vi "Repartidor_colores.vi"() -> ()   [LabVIEW 2017]
uses:
  <extravilib>/ChannelInstances/Stream-bool/Read With Abort.vi
  <extravilib>/ChannelInstances/Stream-bool/Write With Abort.vi
  <extravilib>/ChannelInstances/Stream-bool/EndpointRead.vi
  <extravilib>/ChannelInstances/Stream-bool/Endpoint.vi
  <extravilib>/ChannelInstances/Stream-bool/Instantiate.vi
  <extravilib>/ChannelInstances/Stream-bool/)Channel.vi
  <resource>/ChannelSupport/_ChannelSupport/WaitIfNeeded.vi
  <extravilib>/ChannelInstances/Stream-bool.lvlib
panel:
  out "A 10":u32[][](array[colorbox])
  out "A 9":u32[][](array[colorbox])
  out "A 8":u32[][](array[colorbox])
  out "A 7":u32[][](array[colorbox])
  out "A 6":u32[][](array[colorbox])
  out "A 5":u32[][](array[colorbox])
  out "A 4":u32[][](array[colorbox])
  out "A 3":u32[][](array[colorbox])
  out "A 2":u32[][](array[colorbox])
  out "A":u32[][](array[colorbox])
  out "Array 4":u32[](array[numeric])
  out "element 2":u32
  in  "stop":bool
  out "element":u32
  out "Color Box":u32(colorbox)
  out "Array 2":u32[](array[colorbox])
  out "Array":u32[][](array[colorbox])
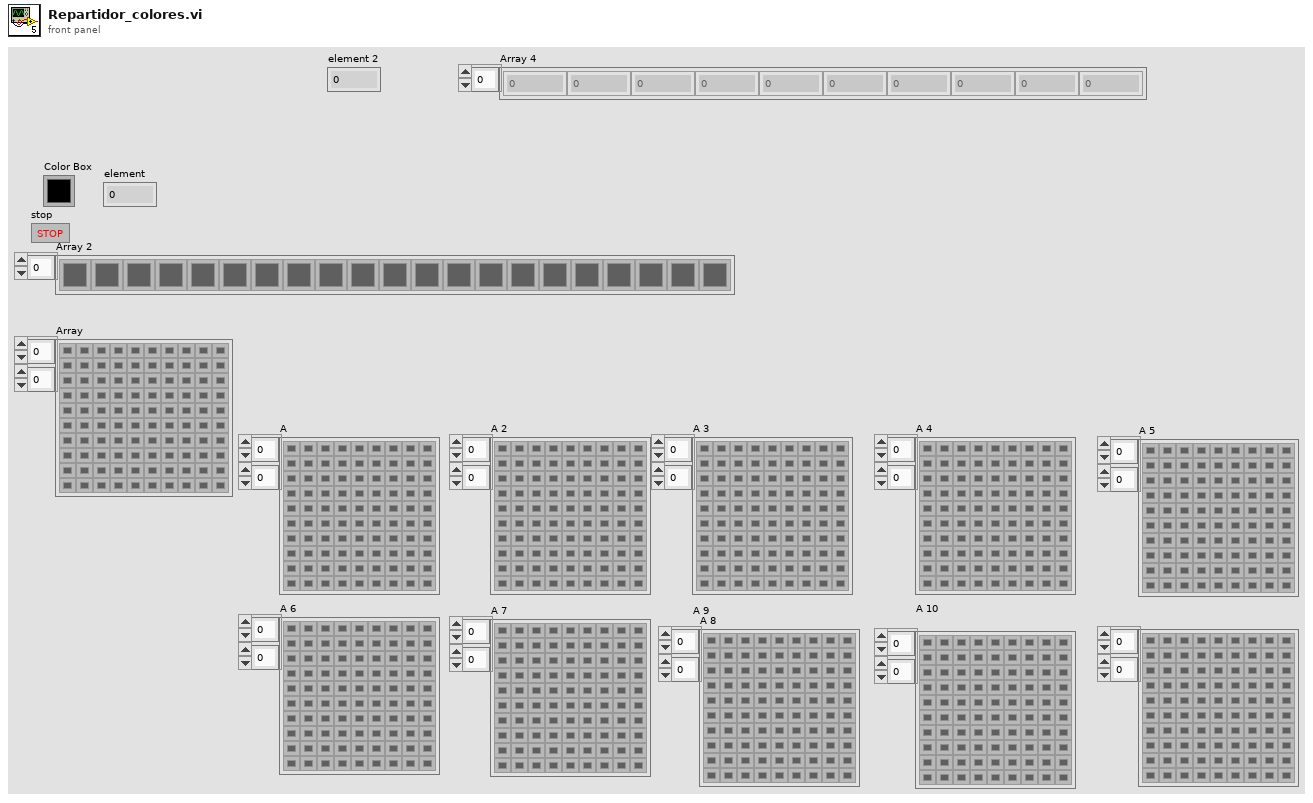
[diagram p1: front panel]
types:
  T1 = cluster{"Numeros":u32[], "A1":u32[], "B1":u32[], "C1":u32[], "D1":u32[], "E1":u32[], "F1":u32[], "G1":u32[], "H1":u32[], "I1":u32[], "J1":u32[]}
  T2 = typedef "Stream-bool.lvlib/)Channel.ctl" = refnum<queue>
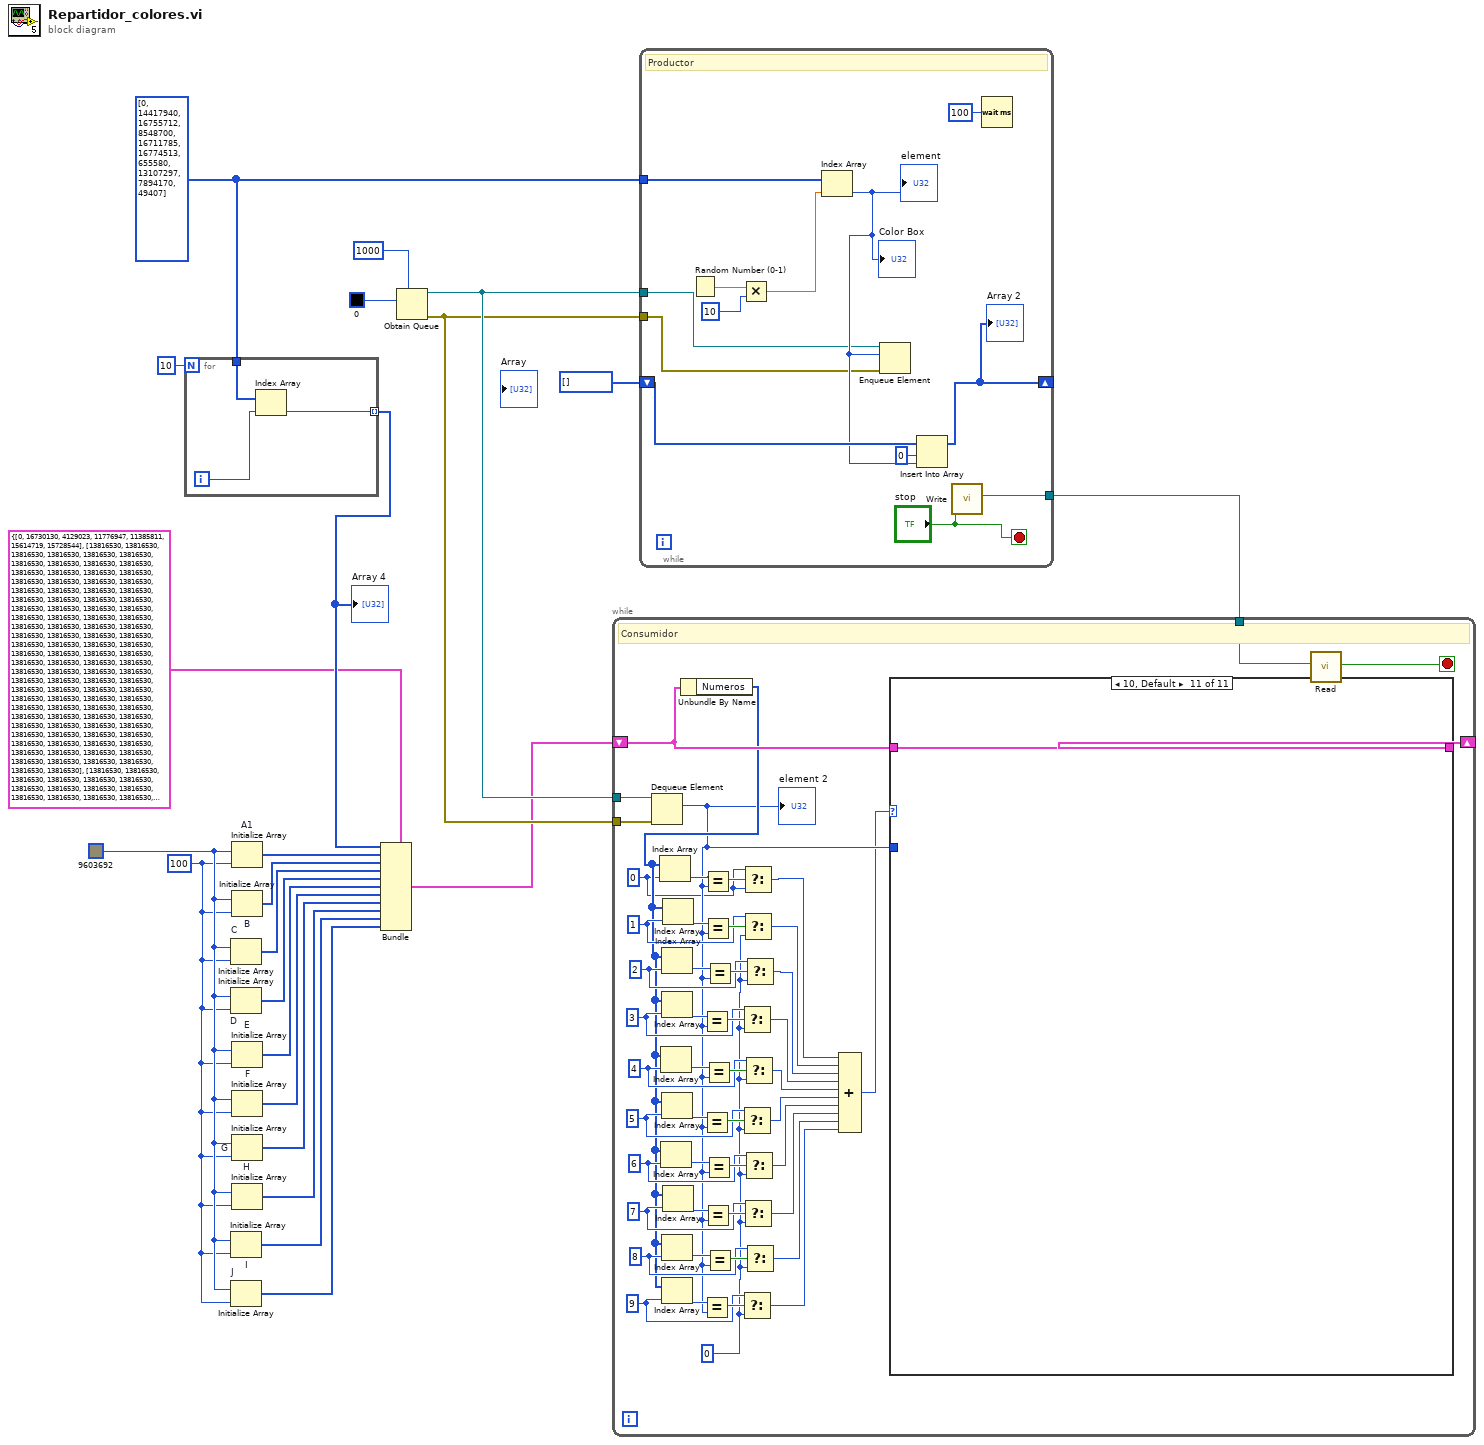
[diagram p0: block diagram]
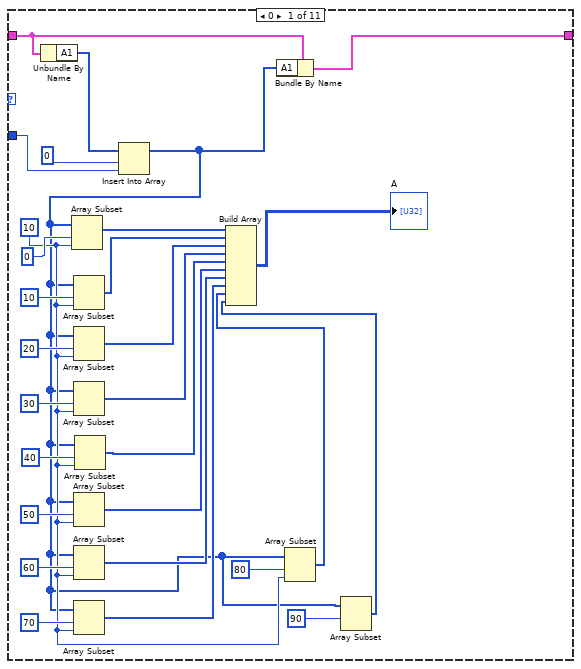
[diagram p2: hidden frame]
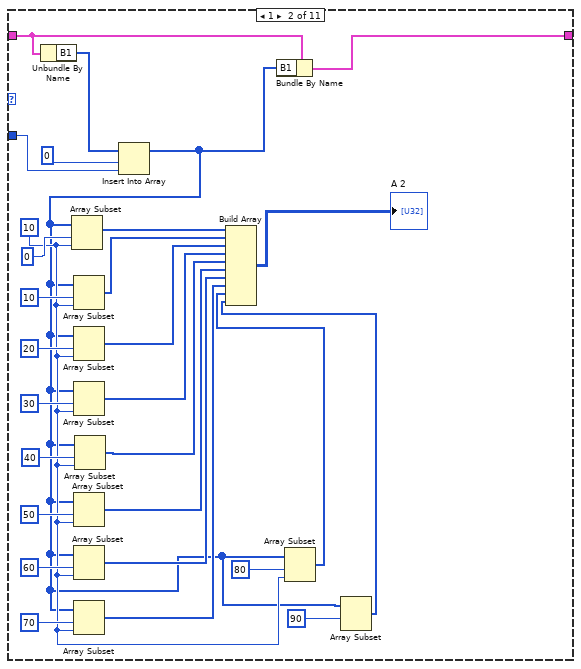
[diagram p3: hidden frame]
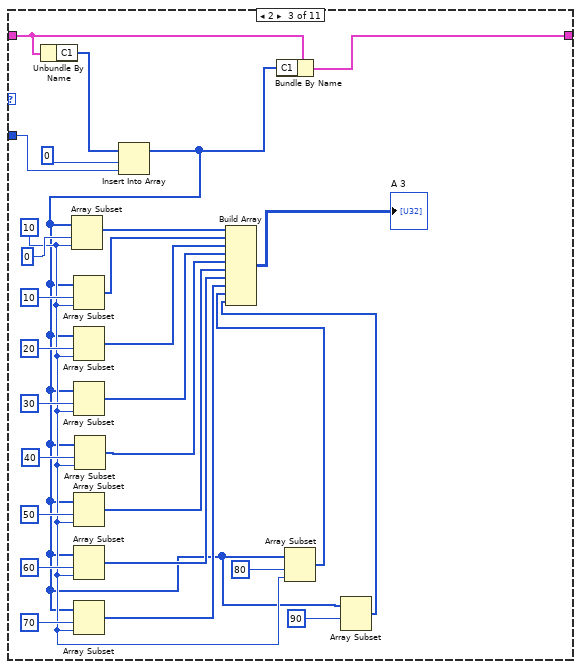
[diagram p4: hidden frame]
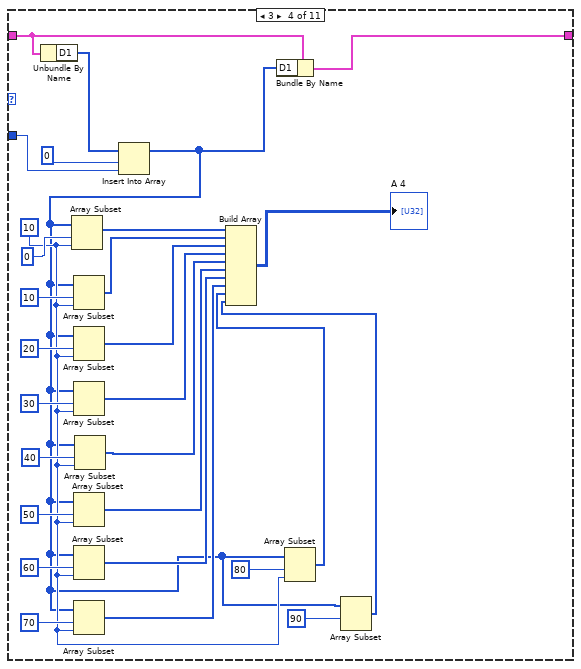
[diagram p5: hidden frame]
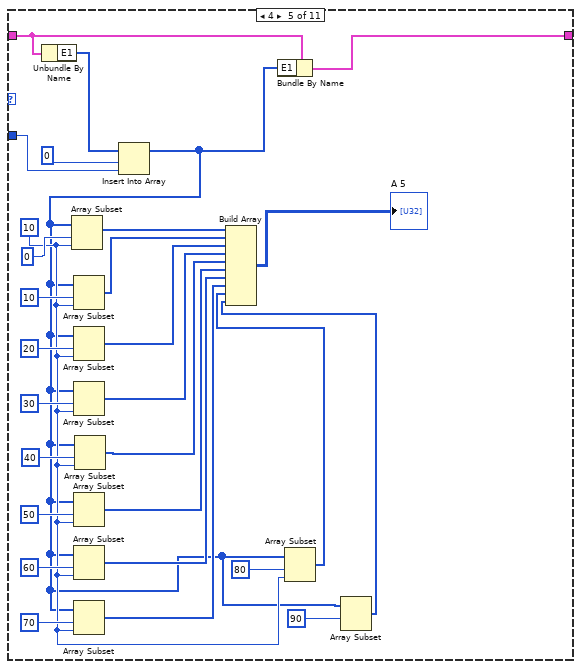
[diagram p6: hidden frame]
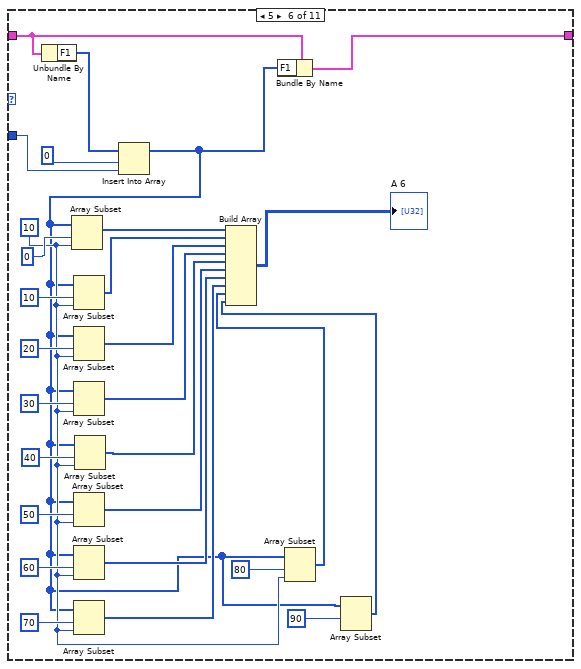
[diagram p7: hidden frame]
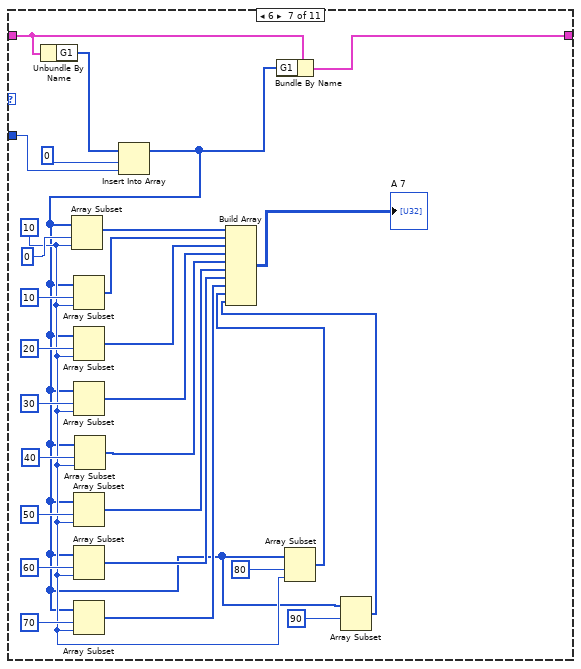
[diagram p8: hidden frame]
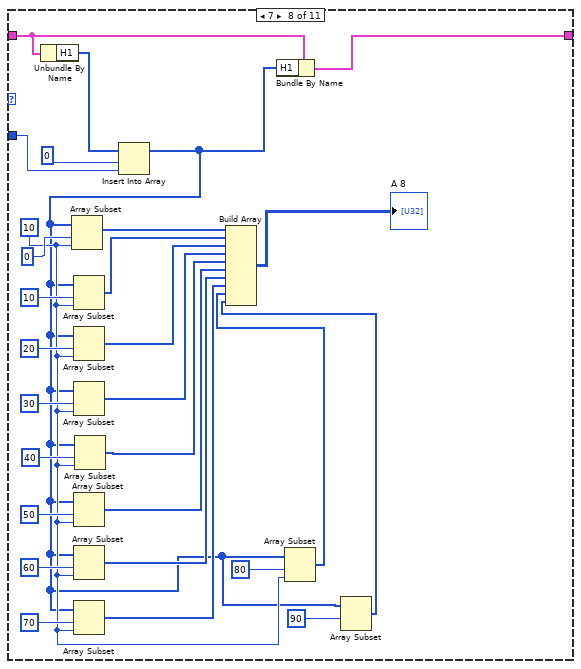
[diagram p9: hidden frame]
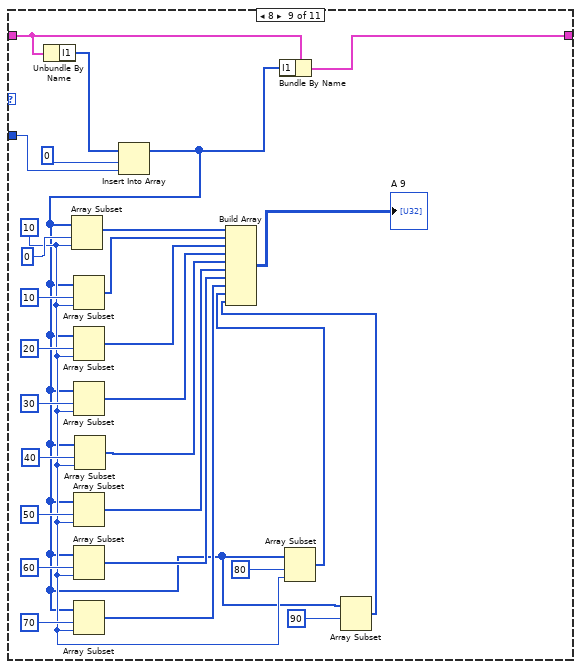
[diagram p10: hidden frame]
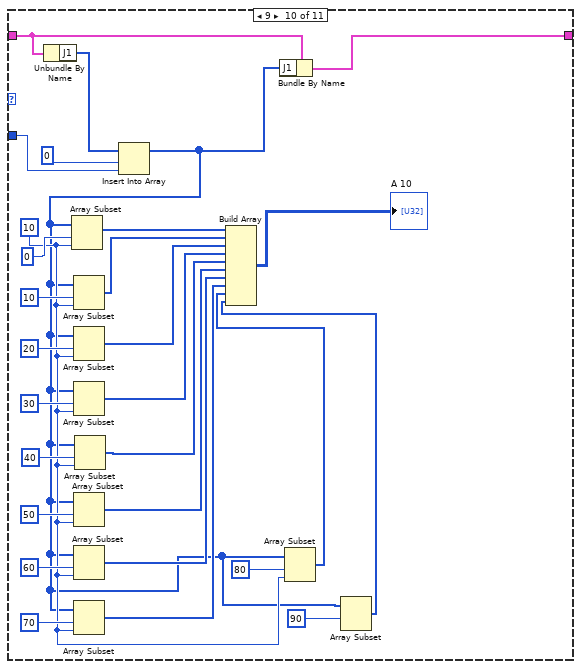
[diagram p11: hidden frame]
diagram:
  w2 = u32[] [0, 14417940, 16755712, 8548700, 16711785, 16774513, 655580, 13107297, 7894170, 49407]
  w18 = u32 9603692
  w17 = 100 ("dimension size")
  n1 = for {
    N: 10 -> [_]
    tunnel: w2 -> [w26]
    tunnel: [w24] -> w7 mode=indexing
    i -> [w25]
    n2 = Index Array "Index Array"(array=w26, index=w25) -> (element=w24:u32)
  }
  "Array 4" <- w7
  n3 = Initialize Array "C"(w18, w17) -> (w16:u32[])
  n4 = Initialize Array "D"(w18, w17) -> (w15:u32[])
  n5 = Initialize Array "I"(w18, w17) -> (w10:u32[])
  n6 = Initialize Array "J"(w18, w17) -> (w9:u32[])
  n7 = Initialize Array "A1"(w18, w17) -> (w5:u32[])
  n8 = Initialize Array "B"(w18, w17) -> (w6:u32[])
  n9 = Initialize Array "E"(w18, w17) -> (w14:u32[])
  n10 = Initialize Array "F"(w18, w17) -> (w13:u32[])
  n11 = Initialize Array "G"(w18, w17) -> (w12:u32[])
  n12 = Initialize Array "H"(w18, w17) -> (w11:u32[])
  n13 = Bundle "Bundle"(cluster=T1 {"Numeros"=[0, 16730130, 4129023, 11776947, 11385811, 15614719, 15728544], "A1"=[13816530, 13816530, 13816530, 13816530, 13816530, 13816530, 13816530, 13816530, 13816530, 13816530, 13816530, 13816530, 13816530, 13816530, 13816530, 13816530, 13816530, 13816530, 13816530, 13816530, 13816530, 13816530, 13816530, 13816530, 13816530, 13816530, 13816530, 13816530, 13816530, 13816530, 13816530, 13816530, 13816530, 13816530, 13816530, 13816530, 13816530, 13816530, 13816530, 13816530, 13816530, 13816530, 13816530, 13816530, 13816530, 13816530, 13816530, 13816530, 13816530, 13816530, 13816530, 13816530, 13816530, 13816530, 13816530, 13816530, 13816530, 13816530, 13816530, 13816530, 13816530, 13816530, 13816530, 13816530, 13816530, 13816530, 13816530, 13816530, 13816530, 13816530, 13816530, 13816530, 13816530, 13816530, 13816530, 13816530, 13816530, 13816530, 13816530, 13816530, 13816530, 13816530, 13816530, 13816530, 13816530, 13816530, 13816530, 13816530, 13816530, 13816530, 13816530, 13816530, 13816530, 13816530, 13816530, 13816530, 13816530, 13816530, 13816530, 13816530], "B1"=[13816530, 13816530, 13816530, 13816530, 13816530, 13816530, 13816530, 13816530, 13816530, 13816530, 13816530, 13816530, 13816530, 13816530, 13816530, 13816530, 13816530, 13816530, 13816530, 13816530, 13816530, 13816530, 13816530, 13816530, 13816530, 13816530, 13816530, 13816530, 13816530, 13816530, 13816530, 13816530, 13816530, 13816530, 13816530, 13816530, 13816530, 13816530, 13816530, 13816530, 13816530, 13816530, 13816530, 13816530, 13816530, 13816530, 13816530, 13816530, 13816530, 13816530, 13816530, 13816530, 13816530, 13816530, 13816530, 13816530, 13816530, 13816530, 13816530, 13816530, 13816530, 13816530, 13816530, 13816530, 13816530, 13816530, 13816530, 13816530, 13816530, 13816530, 13816530, 13816530, 13816530, 13816530, 13816530, 13816530, 13816530, 13816530, 13816530, 13816530, 13816530, 13816530, 13816530, 13816530, 13816530, 13816530, 13816530, 13816530, 13816530, 13816530, 13816530, 13816530, 13816530, 13816530, 13816530, 13816530, 13816530, 13816530, 13816530, 13816530], "C1"=[13816530, 13816530, 13816530, 13816530, 13816530, 13816530, 13816530, 13816530, 13816530, 13816530, 13816530, 13816530, 13816530, 13816530, 13816530, 13816530, 13816530, 13816530, 13816530, 13816530, 13816530, 13816530, 13816530, 13816530, 13816530, 13816530, 13816530, 13816530, 13816530, 13816530, 13816530, 13816530, 13816530, 13816530, 13816530, 13816530, 13816530, 13816530, 13816530, 13816530, 13816530, 13816530, 13816530, 13816530, 13816530, 13816530, 13816530, 13816530, 13816530, 13816530, 13816530, 13816530, 13816530, 13816530, 13816530, 13816530, 13816530, 13816530, 13816530, 13816530, 13816530, 13816530, 13816530, 13816530, 13816530, 13816530, 13816530, 13816530, 13816530, 13816530, 13816530, 13816530, 13816530, 13816530, 13816530, 13816530, 13816530, 13816530, 13816530, 13816530, 13816530, 13816530, 13816530, 13816530, 13816530, 13816530, 13816530, 13816530, 13816530, 13816530, 13816530, 13816530, 13816530, 13816530, 13816530, 13816530, 13816530, 13816530, 13816530, 13816530], "D1"=[13816530, 13816530, 13816530, 13816530, 13816530, 13816530, 13816530, 13816530, 13816530, 13816530, 13816530, 13816530, 13816530, 13816530, 13816530, 13816530, 13816530, 13816530, 13816530, 13816530, 13816530, 13816530, 13816530, 13816530, 13816530, 13816530, 13816530, 13816530, 13816530, 13816530, 13816530, 13816530, 13816530, 13816530, 13816530, 13816530, 13816530, 13816530, 13816530, 13816530, 13816530, 13816530, 13816530, 13816530, 13816530, 13816530, 13816530, 13816530, 13816530, 13816530, 13816530, 13816530, 13816530, 13816530, 13816530, 13816530, 13816530, 13816530, 13816530, 13816530, 13816530, 13816530, 13816530, 13816530, 13816530, 13816530, 13816530, 13816530, 13816530, 13816530, 13816530, 13816530, 13816530, 13816530, 13816530, 13816530, 13816530, 13816530, 13816530, 13816530, 13816530, 13816530, 13816530, 13816530, 13816530, 13816530, 13816530, 13816530, 13816530, 13816530, 13816530, 13816530, 13816530, 13816530, 13816530, 13816530, 13816530, 13816530, 13816530, 13816530], "E1"=[13816530, 13816530, 13816530, 13816530, 13816530, 13816530, 13816530, 13816530, 13816530, 13816530, 13816530, 13816530, 13816530, 13816530, 13816530, 13816530, 13816530, 13816530, 13816530, 13816530, 13816530, 13816530, 13816530, 13816530, 13816530, 13816530, 13816530, 13816530, 13816530, 13816530, 13816530, 13816530, 13816530, 13816530, 13816530, 13816530, 13816530, 13816530, 13816530, 13816530, 13816530, 13816530, 13816530, 13816530, 13816530, 13816530, 13816530, 13816530, 13816530, 13816530, 13816530, 13816530, 13816530, 13816530, 13816530, 13816530, 13816530, 13816530, 13816530, 13816530, 13816530, 13816530, 13816530, 13816530, 13816530, 13816530, 13816530, 13816530, 13816530, 13816530, 13816530, 13816530, 13816530, 13816530, 13816530, 13816530, 13816530, 13816530, 13816530, 13816530, 13816530, 13816530, 13816530, 13816530, 13816530, 13816530, 13816530, 13816530, 13816530, 13816530, 13816530, 13816530, 13816530, 13816530, 13816530, 13816530, 13816530, 13816530, 13816530, 13816530], "F1"=[13816530, 13816530, 13816530, 13816530, 13816530, 13816530, 13816530, 13816530, 13816530, 13816530, 13816530, 13816530, 13816530, 13816530, 13816530, 13816530, 13816530, 13816530, 13816530, 13816530, 13816530, 13816530, 13816530, 13816530, 13816530, 13816530, 13816530, 13816530, 13816530, 13816530, 13816530, 13816530, 13816530, 13816530, 13816530, 13816530, 13816530, 13816530, 13816530, 13816530, 13816530, 13816530, 13816530, 13816530, 13816530, 13816530, 13816530, 13816530, 13816530, 13816530, 13816530, 13816530, 13816530, 13816530, 13816530, 13816530, 13816530, 13816530, 13816530, 13816530, 13816530, 13816530, 13816530, 13816530, 13816530, 13816530, 13816530, 13816530, 13816530, 13816530, 13816530, 13816530, 13816530, 13816530, 13816530, 13816530, 13816530, 13816530, 13816530, 13816530, 13816530, 13816530, 13816530, 13816530, 13816530, 13816530, 13816530, 13816530, 13816530, 13816530, 13816530, 13816530, 13816530, 13816530, 13816530, 13816530, 13816530, 13816530, 13816530, 13816530], "G1"=[13816530, 13816530, 13816530, 13816530, 13816530, 13816530, 13816530, 13816530, 13816530, 13816530, 13816530, 13816530, 13816530, 13816530, 13816530, 13816530, 13816530, 13816530, 13816530, 13816530, 13816530, 13816530, 13816530, 13816530, 13816530, 13816530, 13816530, 13816530, 13816530, 13816530, 13816530, 13816530, 13816530, 13816530, 13816530, 13816530, 13816530, 13816530, 13816530, 13816530, 13816530, 13816530, 13816530, 13816530, 13816530, 13816530, 13816530, 13816530, 13816530, 13816530, 13816530, 13816530, 13816530, 13816530, 13816530, 13816530, 13816530, 13816530, 13816530, 13816530, 13816530, 13816530, 13816530, 13816530, 13816530, 13816530, 13816530, 13816530, 13816530, 13816530, 13816530, 13816530, 13816530, 13816530, 13816530, 13816530, 13816530, 13816530, 13816530, 13816530, 13816530, 13816530, 13816530, 13816530, 13816530, 13816530, 13816530, 13816530, 13816530, 13816530, 13816530, 13816530, 13816530, 13816530, 13816530, 13816530, 13816530, 13816530, 13816530, 13816530], "H1"=[13816530, 13816530, 13816530, 13816530, 13816530, 13816530, 13816530, 13816530, 13816530, 13816530, 13816530, 13816530, 13816530, 13816530, 13816530, 13816530, 13816530, 13816530, 13816530, 13816530, 13816530, 13816530, 13816530, 13816530, 13816530, 13816530, 13816530, 13816530, 13816530, 13816530, 13816530, 13816530, 13816530, 13816530, 13816530, 13816530, 13816530, 13816530, 13816530, 13816530, 13816530, 13816530, 13816530, 13816530, 13816530, 13816530, 13816530, 13816530, 13816530, 13816530, 13816530, 13816530, 13816530, 13816530, 13816530, 13816530, 13816530, 13816530, 13816530, 13816530, 13816530, 13816530, 13816530, 13816530, 13816530, 13816530, 13816530, 13816530, 13816530, 13816530, 13816530, 13816530, 13816530, 13816530, 13816530, 13816530, 13816530, 13816530, 13816530, 13816530, 13816530, 13816530, 13816530, 13816530, 13816530, 13816530, 13816530, 13816530, 13816530, 13816530, 13816530, 13816530, 13816530, 13816530, 13816530, 13816530, 13816530, 13816530, 13816530, 13816530], "I1"=[13816530, 13816530, 13816530, 13816530, 13816530, 13816530, 13816530, 13816530, 13816530, 13816530, 13816530, 13816530, 13816530, 13816530, 13816530, 13816530, 13816530, 13816530, 13816530, 13816530, 13816530, 13816530, 13816530, 13816530, 13816530, 13816530, 13816530, 13816530, 13816530, 13816530, 13816530, 13816530, 13816530, 13816530, 13816530, 13816530, 13816530, 13816530, 13816530, 13816530, 13816530, 13816530, 13816530, 13816530, 13816530, 13816530, 13816530, 13816530, 13816530, 13816530, 13816530, 13816530, 13816530, 13816530, 13816530, 13816530, 13816530, 13816530, 13816530, 13816530, 13816530, 13816530, 13816530, 13816530, 13816530, 13816530, 13816530, 13816530, 13816530, 13816530, 13816530, 13816530, 13816530, 13816530, 13816530, 13816530, 13816530, 13816530, 13816530, 13816530, 13816530, 13816530, 13816530, 13816530, 13816530, 13816530, 13816530, 13816530, 13816530, 13816530, 13816530, 13816530, 13816530, 13816530, 13816530, 13816530, 13816530, 13816530, 13816530, 13816530], "J1"=[13816530, 13816530, 13816530, 13816530, 13816530, 13816530, 13816530, 13816530, 13816530, 13816530, 13816530, 13816530, 13816530, 13816530, 13816530, 13816530, 13816530, 13816530, 13816530, 13816530, 13816530, 13816530, 13816530, 13816530, 13816530, 13816530, 13816530, 13816530, 13816530, 13816530, 13816530, 13816530, 13816530, 13816530, 13816530, 13816530, 13816530, 13816530, 13816530, 13816530, 13816530, 13816530, 13816530, 13816530, 13816530, 13816530, 13816530, 13816530, 13816530, 13816530, 13816530, 13816530, 13816530, 13816530, 13816530, 13816530, 13816530, 13816530, 13816530, 13816530, 13816530, 13816530, 13816530, 13816530, 13816530, 13816530, 13816530, 13816530, 13816530, 13816530, 13816530, 13816530, 13816530, 13816530, 13816530, 13816530, 13816530, 13816530, 13816530, 13816530, 13816530, 13816530, 13816530, 13816530, 13816530, 13816530, 13816530, 13816530, 13816530, 13816530, 13816530, 13816530, 13816530, 13816530, 13816530, 13816530, 13816530, 13816530, 13816530, 13816530]}, "Numeros"=w7, "A1"=w5, "B1"=w6, "C1"=w16, "D1"=w15, "E1"=w14, "F1"=w13, "G1"=w12, "H1"=w11, "I1"=w10, "J1"=w9) -> (w4:T1)
  n14 = Obtain Queue(max queue size (-1, unlimited)=1000, element data type=u32 0) -> (queue out=w20:refnum<queue>, error out=w19:errorcluster)  [unwired: 3 in, 1 out]
  n15 = while {
    shift-right: [w32] -> _
    shift-left: u32[] [] -> [w34]
    tunnel: w19 -> [w30]
    tunnel: w20 -> [w29]
    tunnel: w2 -> [w28]
    tunnel: [w27] -> w1
    stop <- "stop" stop-if-true
    # "Productor"
    n16 = Random Number (0-1)() -> (number: 0 to 1=w39:dbl)
    n17 = Multiply(x=w39, y=10) -> (x*y=w37:dbl)
    n18 = Index Array "Index Array"(array=w28, index=w37) -> (element=w31:u32)
    "element" <- w31
    "Color Box" <- w31
    n19 = Enqueue Element(queue=w29, element=w31, error in (no error)=w30) -> ()  [unwired: 1 in, 3 out]
    n20 = Insert Into Array "Insert Into Array"(array=w34, index=0, new element=w31) -> (w32:u32[])
    "Array 2" <- w32
    n21 = call <extravilib>:"Write.vi"("element"="stop") -> ("channel"=w27:T2)  [unwired: 8 in, 2 out]
    n22 = Wait (ms)(milliseconds to wait=u32 100) -> ()  [unwired: 1 out]
  }
  n23 = while {
    tunnel: w20 -> [w89]
    tunnel: w19 -> [w88]
    shift-right: [w87] -> _
    shift-left: w4 -> [w86]
    tunnel: w1 -> [w41]
    stop <- w40 stop-if-true
    w43 = 0 ("f")
    w66 = 9 ("index")
    w68 = 8 ("index")
    w70 = 7 ("index")
    w72 = 6 ("index")
    w74 = 5 ("index")
    w76 = 4 ("index")
    w78 = 3 ("index")
    w80 = 2 ("index")
    w82 = 1 ("index")
    w54 = 0 ("index")
    # "Consumidor"
    n24 = Dequeue Element(queue=w89, error in (no error)=w88) -> (element=w55:u32)  [unwired: 1 in, 3 out]
    "element 2" <- w55
    n25 = Unbundle By Name(w86) -> ("Numeros"=w65:u32[])
    n26 = Index Array(array=w65, index=w54) -> (element=w85:u32)
    n27 = Index Array(array=w65, index=w76) -> (element=w59:u32)
    n28 = Index Array(array=w65, index=w72) -> (element=w61:u32)
    n29 = Index Array(array=w65, index=w80) -> (element=w57:u32)
    n30 = Index Array(array=w65, index=w78) -> (element=w58:u32)
    n31 = Index Array(array=w65, index=w74) -> (element=w60:u32)
    n32 = Index Array(array=w65, index=w68) -> (element=w63:u32)
    n33 = Index Array(array=w65, index=w66) -> (element=w64:u32)
    n34 = Index Array(array=w65, index=w82) -> (element=w56:u32)
    n35 = Index Array(array=w65, index=w70) -> (element=w62:u32)
    n36 = Equal?(x=w58, y=w55) -> (x = y?=w79:bool)
    n37 = Equal?(x=w60, y=w55) -> (x = y?=w75:bool)
    n38 = Equal?(x=w64, y=w55) -> (x = y?=w67:bool)
    n39 = Equal?(x=w85, y=w55) -> (x = y?=w84:bool)
    n40 = Equal?(x=w56, y=w55) -> (x = y?=w83:bool)
    n41 = Equal?(x=w62, y=w55) -> (x = y?=w71:bool)
    n42 = Equal?(x=w59, y=w55) -> (x = y?=w77:bool)
    n43 = Equal?(x=w61, y=w55) -> (x = y?=w73:bool)
    n44 = Equal?(x=w57, y=w55) -> (x = y?=w81:bool)
    n45 = Equal?(x=w63, y=w55) -> (x = y?=w69:bool)
    n46 = Select(t=w78, s=w79, f=w43) -> (s? t:f=w50:i32)
    n47 = Select(t=w74, s=w75, f=w43) -> (s? t:f=w48:i32)
    n48 = Select(t=w66, s=w67, f=w43) -> (s? t:f=w44:i32)
    n49 = Select(t=w54, s=w84, f=w54) -> (s? t:f=w53:i32)
    n50 = Select(t=w82, s=w83, f=w43) -> (s? t:f=w52:i32)
    n51 = Select(t=w70, s=w71, f=w43) -> (s? t:f=w46:i32)
    n52 = Select(t=w76, s=w77, f=w43) -> (s? t:f=w49:i32)
    n53 = Select(t=w72, s=w73, f=w43) -> (s? t:f=w47:i32)
    n54 = Select(t=w80, s=w81, f=w43) -> (s? t:f=w51:i32)
    n55 = Select(t=w68, s=w69, f=w43) -> (s? t:f=w45:i32)
    n56 = Compound Arithmetic op=ADD(w53, w52, w51, w50, w49, w48, w47, w46, w45, w44) -> (w42:i32)
    n57 = case shown="10, Default" w42 {
      tunnel: w86 -> [w113 w141 w169 w197 w225 w253 w281 w309 w337 w365 w370]
      tunnel: [w115 w143 w171 w199 w227 w255 w283 w311 w339 w367 w370] -> w87
      tunnel: w55 -> [w114 w142 w170 w198 w226 w254 w282 w310 w338 w366 _]
      frame 0 {
        w100 = 10 ("length")
        n58 = Unbundle By Name(w113) -> ("A1"=w116:u32[])
        n59 = Insert Into Array "Insert Into Array"(array=w116, index=0, new element=w114) -> (w91:u32[])
        n60 = Array Subset "Array Subset"(array=w91, index=0 ("length"), length=w100) -> (w112:u32[])
        n61 = Array Subset "Array Subset"(array=w91, index=10, length=w100) -> (w110:u32[])
        n62 = Array Subset "Array Subset"(array=w91, index=20, length=w100) -> (w99:u32[])
        n63 = Array Subset "Array Subset"(array=w91, index=30, length=w100) -> (w98:u32[])
        n64 = Array Subset "Array Subset"(array=w91, index=50, length=w100) -> (w96:u32[])
        n65 = Array Subset "Array Subset"(array=w91, index=60, length=w100) -> (w95:u32[])
        n66 = Array Subset "Array Subset"(array=w91, index=70, length=w100) -> (w94:u32[])
        n67 = Array Subset "Array Subset"(array=w91, index=40, length=w100) -> (w97:u32[])
        n68 = Bundle By Name(cluster=w113, "A1"=w91) -> (w115:T1)
        n69 = Array Subset "Array Subset"(array=w91, index=80, length=w100) -> (w93:u32[])
        n70 = Array Subset "Array Subset"(array=w91, index=90) -> (w90:u32[])  [unwired: 1 in]
        n71 = Build Array(w112, w110, w99, w98, w97, w96, w95, w94, w93, w90) -> (→"A":u32[][])
      }
      frame 1 {
        w128 = 10 ("length")
        n72 = Unbundle By Name(w141) -> ("B1"=w144:u32[])
        n73 = Insert Into Array "Insert Into Array"(array=w144, index=0, new element=w142) -> (w119:u32[])
        n74 = Array Subset "Array Subset"(array=w119, index=0 ("length"), length=w128) -> (w140:u32[])
        n75 = Array Subset "Array Subset"(array=w119, index=10, length=w128) -> (w138:u32[])
        n76 = Array Subset "Array Subset"(array=w119, index=20, length=w128) -> (w127:u32[])
        n77 = Array Subset "Array Subset"(array=w119, index=30, length=w128) -> (w126:u32[])
        n78 = Array Subset "Array Subset"(array=w119, index=50, length=w128) -> (w124:u32[])
        n79 = Array Subset "Array Subset"(array=w119, index=60, length=w128) -> (w123:u32[])
        n80 = Array Subset "Array Subset"(array=w119, index=70, length=w128) -> (w122:u32[])
        n81 = Array Subset "Array Subset"(array=w119, index=40, length=w128) -> (w125:u32[])
        n82 = Bundle By Name(cluster=w141, "B1"=w119) -> (w143:T1)
        n83 = Array Subset "Array Subset"(array=w119, index=80, length=w128) -> (w121:u32[])
        n84 = Array Subset "Array Subset"(array=w119, index=90) -> (w118:u32[])  [unwired: 1 in]
        n85 = Build Array(w140, w138, w127, w126, w125, w124, w123, w122, w121, w118) -> (→"A 2":u32[][])
      }
      frame 2 {
        w156 = 10 ("length")
        n86 = Unbundle By Name(w169) -> ("C1"=w172:u32[])
        n87 = Insert Into Array "Insert Into Array"(array=w172, index=0, new element=w170) -> (w147:u32[])
        n88 = Array Subset "Array Subset"(array=w147, index=0 ("length"), length=w156) -> (w168:u32[])
        n89 = Array Subset "Array Subset"(array=w147, index=10, length=w156) -> (w166:u32[])
        n90 = Array Subset "Array Subset"(array=w147, index=20, length=w156) -> (w155:u32[])
        n91 = Array Subset "Array Subset"(array=w147, index=30, length=w156) -> (w154:u32[])
        n92 = Array Subset "Array Subset"(array=w147, index=50, length=w156) -> (w152:u32[])
        n93 = Array Subset "Array Subset"(array=w147, index=60, length=w156) -> (w151:u32[])
        n94 = Array Subset "Array Subset"(array=w147, index=70, length=w156) -> (w150:u32[])
        n95 = Array Subset "Array Subset"(array=w147, index=40, length=w156) -> (w153:u32[])
        n96 = Bundle By Name(cluster=w169, "C1"=w147) -> (w171:T1)
        n97 = Array Subset "Array Subset"(array=w147, index=80, length=w156) -> (w149:u32[])
        n98 = Array Subset "Array Subset"(array=w147, index=90) -> (w146:u32[])  [unwired: 1 in]
        n99 = Build Array(w168, w166, w155, w154, w153, w152, w151, w150, w149, w146) -> (→"A 3":u32[][])
      }
      frame 3 {
        w184 = 10 ("length")
        n100 = Unbundle By Name(w197) -> ("D1"=w200:u32[])
        n101 = Insert Into Array "Insert Into Array"(array=w200, index=0, new element=w198) -> (w175:u32[])
        n102 = Array Subset "Array Subset"(array=w175, index=0 ("length"), length=w184) -> (w196:u32[])
        n103 = Array Subset "Array Subset"(array=w175, index=10, length=w184) -> (w194:u32[])
        n104 = Array Subset "Array Subset"(array=w175, index=20, length=w184) -> (w183:u32[])
        n105 = Array Subset "Array Subset"(array=w175, index=30, length=w184) -> (w182:u32[])
        n106 = Array Subset "Array Subset"(array=w175, index=50, length=w184) -> (w180:u32[])
        n107 = Array Subset "Array Subset"(array=w175, index=60, length=w184) -> (w179:u32[])
        n108 = Array Subset "Array Subset"(array=w175, index=70, length=w184) -> (w178:u32[])
        n109 = Array Subset "Array Subset"(array=w175, index=40, length=w184) -> (w181:u32[])
        n110 = Bundle By Name(cluster=w197, "D1"=w175) -> (w199:T1)
        n111 = Array Subset "Array Subset"(array=w175, index=80, length=w184) -> (w177:u32[])
        n112 = Array Subset "Array Subset"(array=w175, index=90) -> (w174:u32[])  [unwired: 1 in]
        n113 = Build Array(w196, w194, w183, w182, w181, w180, w179, w178, w177, w174) -> (→"A 4":u32[][])
      }
      frame 4 {
        w212 = 10 ("length")
        n114 = Unbundle By Name(w225) -> ("E1"=w228:u32[])
        n115 = Insert Into Array "Insert Into Array"(array=w228, index=0, new element=w226) -> (w203:u32[])
        n116 = Array Subset "Array Subset"(array=w203, index=0 ("length"), length=w212) -> (w224:u32[])
        n117 = Array Subset "Array Subset"(array=w203, index=10, length=w212) -> (w222:u32[])
        n118 = Array Subset "Array Subset"(array=w203, index=20, length=w212) -> (w211:u32[])
        n119 = Array Subset "Array Subset"(array=w203, index=30, length=w212) -> (w210:u32[])
        n120 = Array Subset "Array Subset"(array=w203, index=50, length=w212) -> (w208:u32[])
        n121 = Array Subset "Array Subset"(array=w203, index=60, length=w212) -> (w207:u32[])
        n122 = Array Subset "Array Subset"(array=w203, index=70, length=w212) -> (w206:u32[])
        n123 = Array Subset "Array Subset"(array=w203, index=40, length=w212) -> (w209:u32[])
        n124 = Bundle By Name(cluster=w225, "E1"=w203) -> (w227:T1)
        n125 = Array Subset "Array Subset"(array=w203, index=80, length=w212) -> (w205:u32[])
        n126 = Array Subset "Array Subset"(array=w203, index=90) -> (w202:u32[])  [unwired: 1 in]
        n127 = Build Array(w224, w222, w211, w210, w209, w208, w207, w206, w205, w202) -> (→"A 5":u32[][])
      }
      frame 5 {
        w240 = 10 ("length")
        n128 = Unbundle By Name(w253) -> ("F1"=w256:u32[])
        n129 = Insert Into Array "Insert Into Array"(array=w256, index=0, new element=w254) -> (w231:u32[])
        n130 = Array Subset "Array Subset"(array=w231, index=0 ("length"), length=w240) -> (w252:u32[])
        n131 = Array Subset "Array Subset"(array=w231, index=10, length=w240) -> (w250:u32[])
        n132 = Array Subset "Array Subset"(array=w231, index=20, length=w240) -> (w239:u32[])
        n133 = Array Subset "Array Subset"(array=w231, index=30, length=w240) -> (w238:u32[])
        n134 = Array Subset "Array Subset"(array=w231, index=50, length=w240) -> (w236:u32[])
        n135 = Array Subset "Array Subset"(array=w231, index=60, length=w240) -> (w235:u32[])
        n136 = Array Subset "Array Subset"(array=w231, index=70, length=w240) -> (w234:u32[])
        n137 = Array Subset "Array Subset"(array=w231, index=40, length=w240) -> (w237:u32[])
        n138 = Bundle By Name(cluster=w253, "F1"=w231) -> (w255:T1)
        n139 = Array Subset "Array Subset"(array=w231, index=80, length=w240) -> (w233:u32[])
        n140 = Array Subset "Array Subset"(array=w231, index=90) -> (w230:u32[])  [unwired: 1 in]
        n141 = Build Array(w252, w250, w239, w238, w237, w236, w235, w234, w233, w230) -> (→"A 6":u32[][])
      }
      frame 6 {
        w268 = 10 ("length")
        n142 = Unbundle By Name(w281) -> ("G1"=w284:u32[])
        n143 = Insert Into Array "Insert Into Array"(array=w284, index=0, new element=w282) -> (w259:u32[])
        n144 = Array Subset "Array Subset"(array=w259, index=0 ("length"), length=w268) -> (w280:u32[])
        n145 = Array Subset "Array Subset"(array=w259, index=10, length=w268) -> (w278:u32[])
        n146 = Array Subset "Array Subset"(array=w259, index=20, length=w268) -> (w267:u32[])
        n147 = Array Subset "Array Subset"(array=w259, index=30, length=w268) -> (w266:u32[])
        n148 = Array Subset "Array Subset"(array=w259, index=50, length=w268) -> (w264:u32[])
        n149 = Array Subset "Array Subset"(array=w259, index=60, length=w268) -> (w263:u32[])
        n150 = Array Subset "Array Subset"(array=w259, index=70, length=w268) -> (w262:u32[])
        n151 = Array Subset "Array Subset"(array=w259, index=40, length=w268) -> (w265:u32[])
        n152 = Bundle By Name(cluster=w281, "G1"=w259) -> (w283:T1)
        n153 = Array Subset "Array Subset"(array=w259, index=80, length=w268) -> (w261:u32[])
        n154 = Array Subset "Array Subset"(array=w259, index=90) -> (w258:u32[])  [unwired: 1 in]
        n155 = Build Array(w280, w278, w267, w266, w265, w264, w263, w262, w261, w258) -> (→"A 7":u32[][])
      }
      frame 7 {
        w296 = 10 ("length")
        n156 = Unbundle By Name(w309) -> ("H1"=w312:u32[])
        n157 = Insert Into Array "Insert Into Array"(array=w312, index=0, new element=w310) -> (w287:u32[])
        n158 = Array Subset "Array Subset"(array=w287, index=0 ("length"), length=w296) -> (w308:u32[])
        n159 = Array Subset "Array Subset"(array=w287, index=10, length=w296) -> (w306:u32[])
        n160 = Array Subset "Array Subset"(array=w287, index=20, length=w296) -> (w295:u32[])
        n161 = Array Subset "Array Subset"(array=w287, index=30, length=w296) -> (w294:u32[])
        n162 = Array Subset "Array Subset"(array=w287, index=50, length=w296) -> (w292:u32[])
        n163 = Array Subset "Array Subset"(array=w287, index=60, length=w296) -> (w291:u32[])
        n164 = Array Subset "Array Subset"(array=w287, index=70, length=w296) -> (w290:u32[])
        n165 = Array Subset "Array Subset"(array=w287, index=40, length=w296) -> (w293:u32[])
        n166 = Bundle By Name(cluster=w309, "H1"=w287) -> (w311:T1)
        n167 = Array Subset "Array Subset"(array=w287, index=80, length=w296) -> (w289:u32[])
        n168 = Array Subset "Array Subset"(array=w287, index=90) -> (w286:u32[])  [unwired: 1 in]
        n169 = Build Array(w308, w306, w295, w294, w293, w292, w291, w290, w289, w286) -> (→"A 8":u32[][])
      }
      frame 8 {
        w324 = 10 ("length")
        n170 = Unbundle By Name(w337) -> ("I1"=w340:u32[])
        n171 = Insert Into Array "Insert Into Array"(array=w340, index=0, new element=w338) -> (w315:u32[])
        n172 = Array Subset "Array Subset"(array=w315, index=0 ("length"), length=w324) -> (w336:u32[])
        n173 = Array Subset "Array Subset"(array=w315, index=10, length=w324) -> (w334:u32[])
        n174 = Array Subset "Array Subset"(array=w315, index=20, length=w324) -> (w323:u32[])
        n175 = Array Subset "Array Subset"(array=w315, index=30, length=w324) -> (w322:u32[])
        n176 = Array Subset "Array Subset"(array=w315, index=50, length=w324) -> (w320:u32[])
        n177 = Array Subset "Array Subset"(array=w315, index=60, length=w324) -> (w319:u32[])
        n178 = Array Subset "Array Subset"(array=w315, index=70, length=w324) -> (w318:u32[])
        n179 = Array Subset "Array Subset"(array=w315, index=40, length=w324) -> (w321:u32[])
        n180 = Bundle By Name(cluster=w337, "I1"=w315) -> (w339:T1)
        n181 = Array Subset "Array Subset"(array=w315, index=80, length=w324) -> (w317:u32[])
        n182 = Array Subset "Array Subset"(array=w315, index=90) -> (w314:u32[])  [unwired: 1 in]
        n183 = Build Array(w336, w334, w323, w322, w321, w320, w319, w318, w317, w314) -> (→"A 9":u32[][])
      }
      frame 9 {
        w352 = 10 ("length")
        n184 = Unbundle By Name(w365) -> ("J1"=w368:u32[])
        n185 = Insert Into Array "Insert Into Array"(array=w368, index=0, new element=w366) -> (w343:u32[])
        n186 = Array Subset "Array Subset"(array=w343, index=0 ("length"), length=w352) -> (w364:u32[])
        n187 = Array Subset "Array Subset"(array=w343, index=10, length=w352) -> (w362:u32[])
        n188 = Array Subset "Array Subset"(array=w343, index=20, length=w352) -> (w351:u32[])
        n189 = Array Subset "Array Subset"(array=w343, index=30, length=w352) -> (w350:u32[])
        n190 = Array Subset "Array Subset"(array=w343, index=50, length=w352) -> (w348:u32[])
        n191 = Array Subset "Array Subset"(array=w343, index=60, length=w352) -> (w347:u32[])
        n192 = Array Subset "Array Subset"(array=w343, index=70, length=w352) -> (w346:u32[])
        n193 = Array Subset "Array Subset"(array=w343, index=40, length=w352) -> (w349:u32[])
        n194 = Bundle By Name(cluster=w365, "J1"=w343) -> (w367:T1)
        n195 = Array Subset "Array Subset"(array=w343, index=80, length=w352) -> (w345:u32[])
        n196 = Array Subset "Array Subset"(array=w343, index=90) -> (w342:u32[])  [unwired: 1 in]
        n197 = Build Array(w364, w362, w351, w350, w349, w348, w347, w346, w345, w342) -> (→"A 10":u32[][])
      }
      frame 10, Default {
      }
    }
    n198 = call <extravilib>:"Read.vi"("channel"=w41) -> ("element"=w40:bool)  [unwired: 6 in, 4 out]
  }
